vi "_Change Bookmark Image.vi"(7 "Picture Control Reference":refnum<vi>, 8 "error in (no error)":errorcluster, 9 "No Image?":bool, 10 "Bookmark ID":u32, 11 "vi path":path) -> (0 "error out":errorcluster)   [LabVIEW 2017, in "CSM_ExampleBrowser.lvlib"]
uses:
  CSM_ExampleBrowser.lvlib
  <vilib>/Utility/miscctls.llb/LVPointTypeDef.ctl
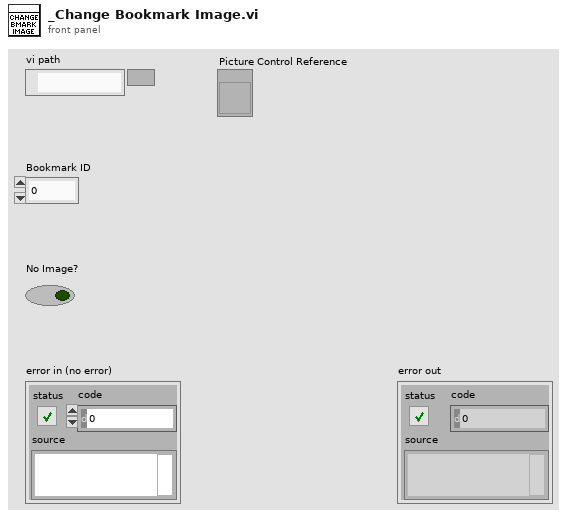
[diagram p1: front panel]
types:
  T1 = typedef "LVPointTypeDef.ctl" = cluster{"Horizontal":i16, "Vertical":i16}
  T2 = cluster{"horizontal":enum16{"left", "center", "right"}, "vertical":enum16{"top", "center", "bottom"}}
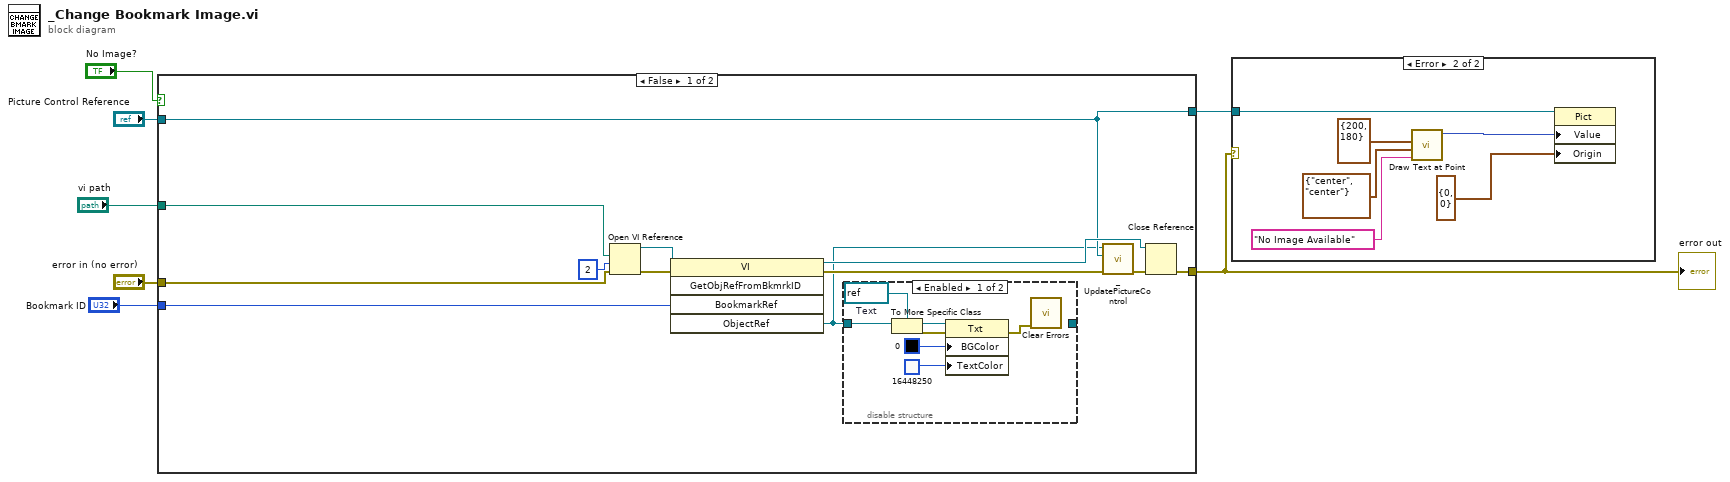
[diagram p0: block diagram]
diagram:
  n1 = case shown="False" "No Image?" {
    tunnel: [w19 w29] -> w2
    tunnel: "error in (no error)" -> [w15 w29]
    tunnel: "Picture Control Reference" -> [w9 w28]
    tunnel: "Bookmark ID" -> [w11 _]
    tunnel: "vi path" -> [w10 _]
    tunnel: [w9 w28] -> w1
    frame False {
      n2 = Open VI Reference(vi path=w10, options=2, error in (no error)=w15) -> (vi reference=w17:refnum<vi>, error out=w18:errorcluster)  [unwired: 3 in]
      n3 = invoke class="VI" method="GetObjRefFromBkmrkID"(reference=w17, error in=w18, "BookmarkRef"=w11) -> (reference out=w16:refnum<vi>, error out=w13:errorcluster, "ObjectRef"=w8:refnum<vi>)  [unwired: 2 in, 2 out]
      n4 = disable-structure shown="Enabled" {
        disable-tunnel: w8 -> [w26 w27]
        disable-tunnel: [_ w27] -> _
        frame Enabled {
          w23 = refnum<vi> refnum  # Text
          n5 = To More Specific Class(target class=w23, reference=w26) -> (specific class reference=w25:refnum<vi>, error out=w22:errorcluster)  [unwired: 1 in]
          n6 = property class="Txt"(reference=w25, error in=w22, "BGColor"=u32 0, "TextColor"=u32 16448250) -> (error out=w24:errorcluster)  [unwired: 1 out]
          n7 = call <vilib>:"Clear Errors.vi"("error in (no error)"=w24) -> ()  [unwired: 5 in, 2 out]
        }
        frame Disabled {
        }
      }
      n8 = call "_UpdatePictureControl.vi"("error in (no error)"=w13, "Picture Control Reference"=w9, "Center Object Reference"=w8) -> ("error out"=w14:errorcluster)  [unwired: 8 in]
      n9 = Close Reference(reference=w16, error in (no error)=w14) -> (error out=w19:errorcluster)
    }
    frame True {
    }
  }
  "error out" <- w2
  n10 = case shown="Error" w2 {
    tunnel: w1 -> [_ w30]
    frame No Error {
    }
    frame Error {
      n11 = call <vilib>:"Draw Text at Point.vi"("text"="No Image Available", "alignment(left, top)"=T2 {"horizontal"=enum."center", "vertical"=enum."center"}, "origin"=cluster{"x":i16, "y":i16} {"x"=200, "y"=180}) -> ("new picture"=w35:picture)  [unwired: 7 in, 1 out]
      n12 = property class="Pict"(reference=w30, "Value"=w35, "Origin"=T1 {"Horizontal"=0, "Vertical"=0}) -> ()  [unwired: 1 in, 2 out]
    }
  }
